vi "settings_filename_from_registry.vi"() -> (2 "Last Used Settings File":string)   [LabVIEW 2010]
uses:
  <vilib>/registry/registry.llb/Registry SAM.ctl
  <vilib>/registry/registry.llb/Registry RtKey.ctl
  <vilib>/registry/registry.llb/Read Registry Value Simple STR.vi
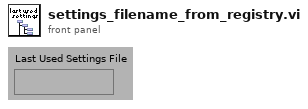
[diagram p1: front panel]
types:
  T1 = typedef "Registry SAM.ctl" = enum32{"KEY_QUERY_VALUE", "KEY_SET_VALUE", "KEY_CREATE_SUB_KEY", "KEY_ENUMERATE_SUB_KEYS", "KEY_NOTIFY", "KEY_CREATE_LINK", "KEY_READ", "KEY_WRITE", "KEY_ALL_ACCESS", "KEY_READ | KEY_WRITE"}
  T2 = typedef "Registry RtKey.ctl" = enum32{"HKEY_CLASSES_ROOT", "HKEY_CURRENT_USER", "HKEY_LOCAL_MACHINE", "HKEY_USERS", "HKEY_PERFORMANCE_DATA", "HKEY_CURRENT_CONFIG", "HKEY_DYN_DATA"}
  T3 = typedef "Registry refnum.ctl" = refnum<k1>
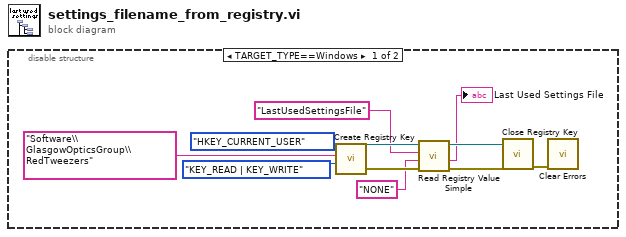
[diagram p0: block diagram]
diagram:
  n1 = disable-structure shown="TARGET_TYPE==Windows" {
    frame condition #0 (active) {
      n2 = call <vilib>:"Create Registry Key.vi"("security access mask (KEY_READ | KEY_WRITE)"=Registry_SAM."KEY_READ | KEY_WRITE", "subkey"="Software\\GlasgowOpticsGroup\\RedTweezers", "root key (HKEY_LOCAL_MACHINE)"=Registry_RtKey."HKEY_CURRENT_USER") -> ("error out"=w8:errorcluster, "refnum out"=w6:T3)  [unwired: 6 in, 1 out]
      n3 = call-poly <vilib>:"Read Registry Value Simple.vi"("error in (no error)"=w8, "default data"="NONE", "value"="LastUsedSettingsFile", "refnum"=w6) -> ("error out"=w7:errorcluster, "String/Binary data"=→"Last Used Settings File":string, "refnum out"=w5:T3)  [unwired: 2 in, 1 out]
      n4 = call <vilib>:"Close Registry Key.vi"("error in (no error)"=w7, "refnum"=w5) -> ("error out"=w1:errorcluster)  [unwired: 5 in]
      n5 = call <vilib>:"Clear Errors.vi"("error in (no error)"=w1) -> ()  [unwired: 6 in, 1 out]
    }
    frame condition #1 {
    }
  }
